vi "Untitled 25 (SubVI).vi"(10 "Data":string, 11 "Data 2":string) -> ()   [LabVIEW 2019]
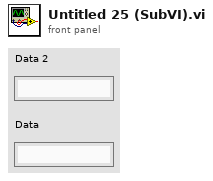
[diagram p1: front panel]
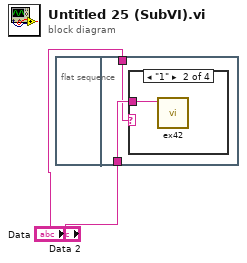
[diagram p0: block diagram]
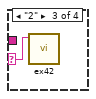
[diagram p3: hidden frame]
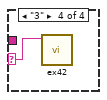
[diagram p4: hidden frame]
diagram:
  n1 = flat-sequence {
    tunnel: "Data 2" -> [w4]
    tunnel: "Data" -> [w3]
    frame #0 {
    }
    frame #1 {
      n2 = case shown="\"1\"" w3 {
        selector: w3 -> [_ _ w6 w7]
        tunnel: w4 -> [_ w5 _ _]
        frame "0", Default {
        }
        frame "1" {
          n3 = call "ex42.vi"("Data"=w5) -> ()  [unwired: 11 in]
        }
        frame "2" {
          n4 = call "ex42.vi"("Data"=w6) -> ()  [unwired: 11 in]
        }
        frame "3" {
          n5 = call "ex42.vi"("Data"=w7) -> ()  [unwired: 11 in]
        }
      }
    }
  }
